vi "Q regex box.vi"(8 "token ?":bool=TRUE, 9 "string":string, 11 "token type":string="number") -> (0 "match ?":bool, 1 "whole match":string, 3 "regexp":string)   [LabVIEW 2015]
uses:
  <vilib>/regexp/Match Regular Expression.xnode
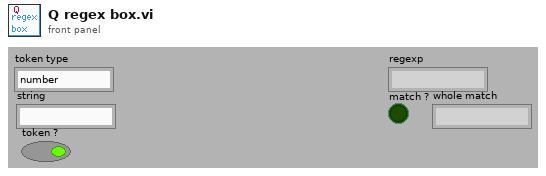
[diagram p1: front panel]
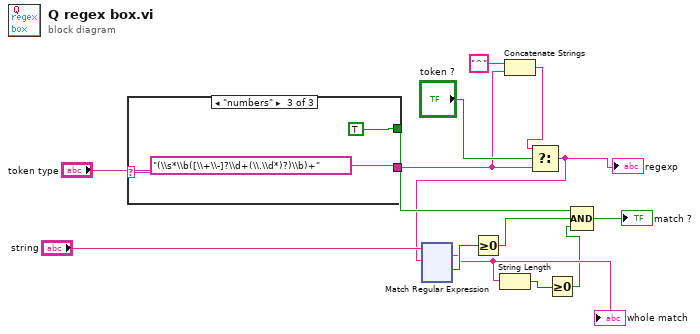
[diagram p0: block diagram]
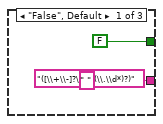
[diagram p2: hidden frame]
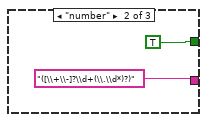
[diagram p3: hidden frame]
diagram:
  n1 = case shown="\"numbers\"" "token type" {
    tunnel: [" " "([\\+\\-]?\\d+(\\.\\d*)?)" "(\\s*\\b([\\+\\-]?\\d+(\\.\\d*)?)\\b)+"] -> w2
    tunnel: [FALSE TRUE TRUE] -> w12
    frame "False", Default {
      (unwired) "([\\+\\-]?\\d+(\\.\\d*)?)"
    }
    frame "number" {
    }
    frame "numbers" {
    }
  }
  n2 = Concatenate Strings("^" ("string"), w2) -> (w4:string)
  n3 = Select(t=w4, s="token ?", f=w2) -> (s? t:f=w1:string)
  "regexp" <- w1
  n4 = xnode "Match Regular Expression"("input string"="string", "regular expression"=w1) -> ("whole match"=w10:string, "offset past match"=w11:i32)  [unwired: 4 in, 3 out]
  "whole match" <- w10
  n5 = Greater Or Equal To 0?(x=w11) -> (x >= 0?=w7:bool)
  n6 = String Length(string=w10) -> (length=w9:i32)
  n7 = Greater Or Equal To 0?(x=w9) -> (x >= 0?=w8:bool)
  n8 = Compound Arithmetic op=AND(w12, w7, w8) -> (→"match ?":bool)
